vi "LN Vector Elements.vi"(11 "Vector (in)":T1=[[2.718], [1.0], [3.0]] format="%_8f") -> (3 "Real Matrix (Column Vector)":T1=[[0.999896315728952], [0.0], [1.0986122886681098]] format="%_8f")   [LabVIEW 2014]
uses:
  <vilib>/Analysis/Matrix/Datatypes/RealMatrix.ctl
  <vilib>/Analysis/Matrix/NI_Matrix.lvlib
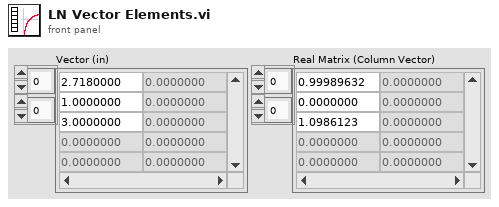
[diagram p1: front panel]
types:
  T1 = typedef "NI_Matrix.lvlib/RealMatrix.ctl" = dbl[][]
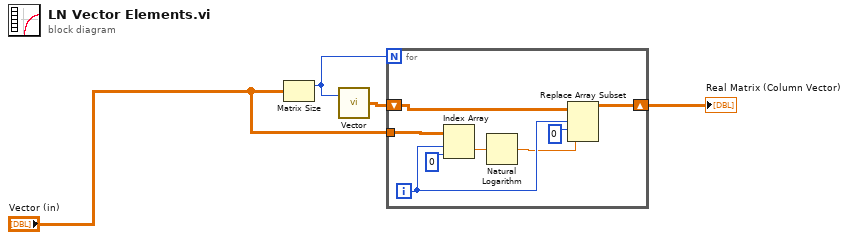
[diagram p0: block diagram]
diagram:
  n1 = Matrix Size(0:"Vector (in)") -> (1:w2:i32)  [unwired: 1 out]
  n2 = call "Vector.vi"("length"=w2) -> ("Real Matrix (Column Vector)"=w3:T1)  [unwired: 1 in]
  n3 = for {
    N: w2 -> [_]
    tunnel: "Vector (in)" -> [w9]
    shift-right: [w11] -> w4
    shift-left: w3 -> [w12]
    i -> [w8]
    n4 = Index Array(array=w9, index (row)=w8, index (col)=0) -> (element=w5:dbl)
    n5 = Natural Logarithm(1:w5) -> (0:w6:dbl)
    n6 = Replace Array Subset(array=w12, new element=w6, index (row)=w8, index (col)=0 ("disabled index (col)")) -> (w11:T1)
  }
  "Real Matrix (Column Vector)" <- w4
